vi "Close.vi"(8 "error in (no error)":errorcluster, 11 "CAN in":refnum<class "CAN.lvclass">) -> (0 "error out":errorcluster, 3 "CAN out":refnum<class "CAN.lvclass">)   [LabVIEW 2019, in "CAN.lvclass"]
uses:
  CAN.lvclass
  CAN.lvclass/CAN.ctl
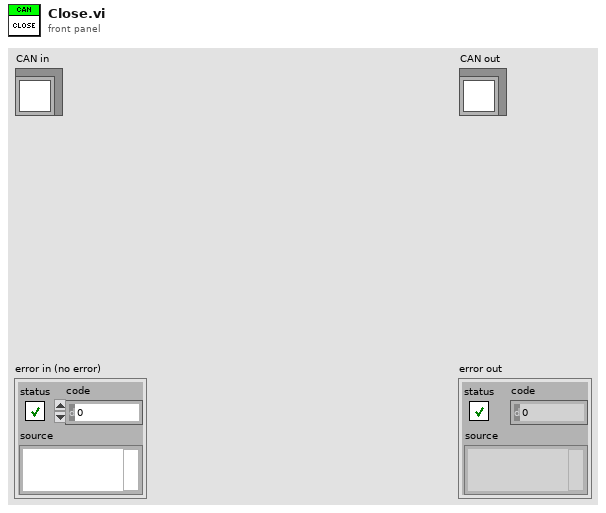
[diagram p1: front panel]
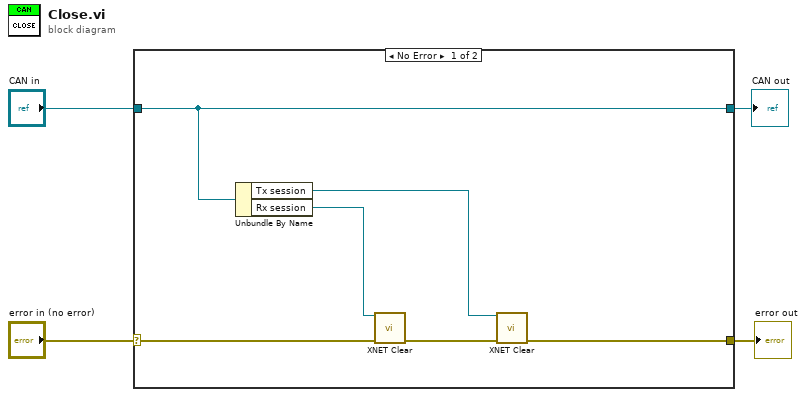
[diagram p0: block diagram]
diagram:
  n1 = case shown="No Error" "error in (no error)" {
    selector: "error in (no error)" -> [w7 w12]
    tunnel: [w6 w12] -> w3
    tunnel: [w5 w11] -> w1
    tunnel: "CAN in" -> [w5 w11]
    frame No Error {
      n2 = Unbundle By Name(w5) -> ("Tx session"=w10:refnum<k21>, "Rx session"=w9:refnum<k21>)
      n3 = call <vilib>:"XNET Clear.vi"("session in"=w9, "error in (no error)"=w7) -> ("error out"=w8:errorcluster)  [unwired: 13 in]
      n4 = call <vilib>:"XNET Clear.vi"("session in"=w10, "error in (no error)"=w8) -> ("error out"=w6:errorcluster)  [unwired: 13 in]
    }
    frame Error {
    }
  }
  "error out" <- w3
  "CAN out" <- w1
